vi "_API_BINANCE_POST_EnableFastWithdrawSwich.vi"(0 "BinanceAPI in":refnum<class "BinanceAPI_.lvclass">, 11 "error in (no error)":errorcluster) -> (4 "BinanceAPI out":refnum<class "BinanceAPI_.lvclass">, 14 "Body":string, 15 "error out":errorcluster)   [LabVIEW 2022 SP3, in "BinanceAPI_.lvclass"]
doc: "https://binance-docs.github.io/apidocs/spot/en/#enable-fast-withdraw-switch-user_data"
uses:
  BinanceAPI_.lvclass
  BinanceAPI_.lvclass/BinanceAPI_.ctl
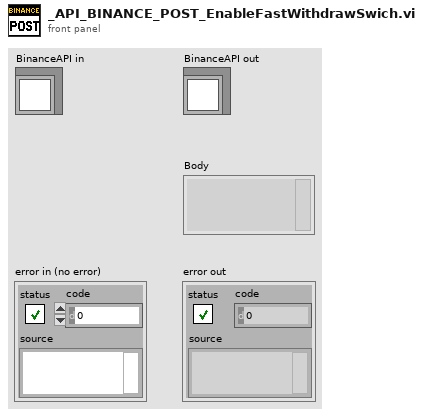
[diagram p1: front panel]
types:
  T1 = enum16{"SPOT", "USDT_FUTURES", "COIN_FUTURES", "VANILLA"}
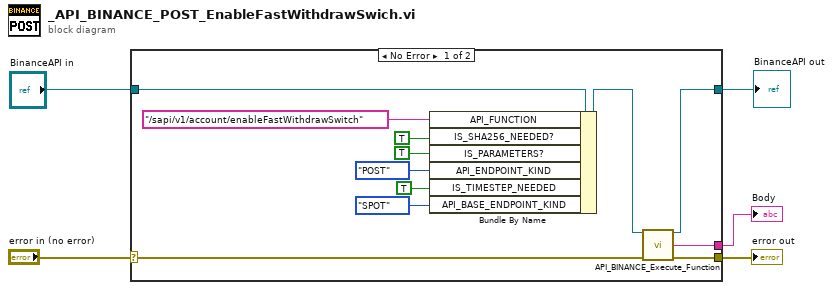
[diagram p0: block diagram]
diagram:
  n1 = case shown="No Error" "error in (no error)" {
    selector: "error in (no error)" -> [w10 w19]
    tunnel: [w9 w19] -> w4
    tunnel: [w11 w18] -> w1
    tunnel: "BinanceAPI in" -> [w13 w18]
    tunnel: [w6 _] -> w3
    frame No Error {
      n2 = Bundle By Name(cluster=w13, "API_FUNCTION"="/sapi/v1/account/enableFastWithdrawSwitch", "IS_SHA256_NEEDED?"=TRUE, "IS_PARAMETERS?"=TRUE, "API_ENDPOINT_KIND"=enum16{"POST", "DELETE", "GET", "PUT"}."POST", "IS_TIMESTEP_NEEDED"=TRUE ("IS_SHA256_NEEDED?"), "API_BASE_ENDPOINT_KIND"=T1."SPOT") -> (w12:refnum<class "BinanceAPI_.lvclass">)
      n3 = call "API_BINANCE_Execute_Function.vi"("BinanceAPI in"=w12, "error in (no error)"=w10) -> ("BinanceAPI out"=w11:refnum<class "BinanceAPI_.lvclass">, "Body"=w6:string, "error out"=w9:errorcluster)  [unwired: 9 in, 2 out]
    }
    frame Error {
    }
  }
  "error out" <- w4
  "Body" <- w3
  "BinanceAPI out" <- w1
